vi "DownloadRuntime.vi"(4 "check version":bool=TRUE, 5 "Path":path, 6 "error in":errorcluster, 9 "WebSocket connection":refnum<k5>) -> (0 "error out":errorcluster, 3 "WebSocket connection out":refnum<k5>)   [LabVIEW 2014, in "RasPiDownloader.lvlib"]
uses:
  RasPiDownloader.lvlib
  Websocket/Websocket.lvlib
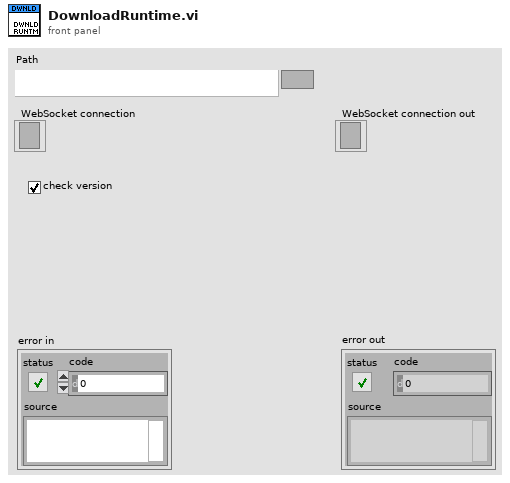
[diagram p1: front panel]
types:
  T1 = typedef "RasPiDownloader.lvlib/RuntimeVersion.ctl" = cluster{"Major":i32, "Minor":i32, "Build":i32, "Revision":i32}
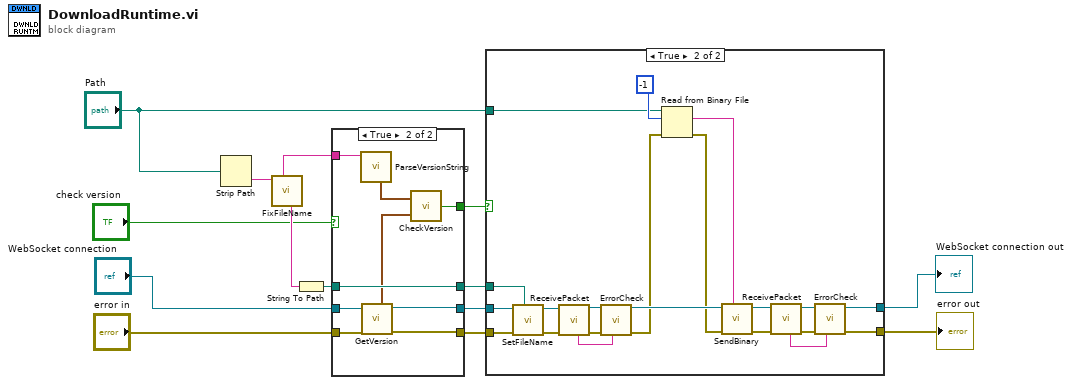
[diagram p0: block diagram]
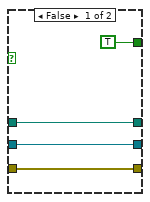
[diagram p2: hidden frame]
diagram:
  n1 = Strip Path(path="Path") -> (name=w11:string)  [unwired: 1 out]
  n2 = call "FixFileName.vi"("Filename"=w11) -> ("fixed filename"=w10:string, "version"=w1:string)  [unwired: 7 in]
  n3 = String To Path(string=w10) -> (path=w8:path)
  n4 = case shown="True" "check version" {
    tunnel: [TRUE w21] -> w9
    tunnel: w8 -> [w17 w22]
    tunnel: [w16 w25] -> w7
    tunnel: "WebSocket connection" -> [w16 w27]
    tunnel: [w15 w24] -> w5
    tunnel: "error in" -> [w15 w26]
    tunnel: [w17 w22] -> w3
    tunnel: w1 -> [_ w23]
    frame False {
    }
    frame True {
      n5 = call "ParseVersionString.vi"("version string"=w23) -> ("Version"=w20:T1)  [unwired: 7 in, 1 out]
      n6 = call "GetVersion.vi"("error in"=w26, "connection ID"=w27) -> ("error out"=w24:errorcluster, "connection ID out"=w25:refnum<k5>, "Version"=w19:T1)  [unwired: 5 in]
      n7 = call "CheckVersion.vi"("Current Version"=w19, "New Version"=w20) -> ("update"=w21:bool)
    }
  }
  n8 = case shown="True" w9 {
    tunnel: w7 -> [w29 w36]
    tunnel: w5 -> [w28 w35]
    tunnel: [w29 w34] -> w14
    tunnel: [w28 w32] -> w13
    tunnel: "Path" -> [_ w31]
    tunnel: w3 -> [_ w30]
    frame False {
    }
    frame True {
      n9 = call "SetFileName.vi"("Path"=w30, "error in"=w35, "WebSocket connection"=w36) -> ("error out"=w48:errorcluster, "WebSocket connection out"=w47:refnum<k5>)  [unwired: 5 in]
      n10 = call "ReceivePacket.vi"("error in"=w48, "connection ID"=w47) -> ("error out"=w40:errorcluster, "connection ID out"=w45:refnum<k5>, "payload"=w37:string)  [unwired: 5 in]
      n11 = call "ErrorCheck.vi"("payload"=w37, "error in"=w40) -> ("error out"=w39:errorcluster)  [unwired: 7 in]
      n12 = Read from Binary File(8:w39, 10:-1 ("count (1)"), 11:w31) -> (0:w44:errorcluster, 2:w43:string)  [unwired: 3 in, 2 out]
      n13 = call "SendBinary.vi"("payload"=w43, "error in"=w44, "connection ID"=w45) -> ("error out"=w42:errorcluster, "connection ID out"=w41:refnum<k5>)  [unwired: 5 in]
      n14 = call "ReceivePacket.vi"("error in"=w42, "connection ID"=w41) -> ("error out"=w38:errorcluster, "connection ID out"=w34:refnum<k5>, "payload"=w33:string)  [unwired: 5 in]
      n15 = call "ErrorCheck.vi"("payload"=w33, "error in"=w38) -> ("error out"=w32:errorcluster)  [unwired: 7 in]
    }
  }
  "WebSocket connection out" <- w14
  "error out" <- w13
